vi "EOL CAN_FBL_S19 C70.vi"(8 "Error in":errorcluster, 10 "Read Session in":refnum<k21>, 11 "Write Session in":refnum<k21>) -> (1 "Motor Calibration Response":string, 2 "debug log":string[][](array[string]), 3 "Response Good?":bool)   [LabVIEW 2018]
uses:
  <vilib>/xnet/xnet.llb/XNET Frame CAN.ctl
  <vilib>/xnet/xnet.llb/XNET Frame Type CAN.ctl
panel:
  out "Rx Data":u8[](array[numeric])
  out "Error out":errorcluster
  in  "Retries":i32=2
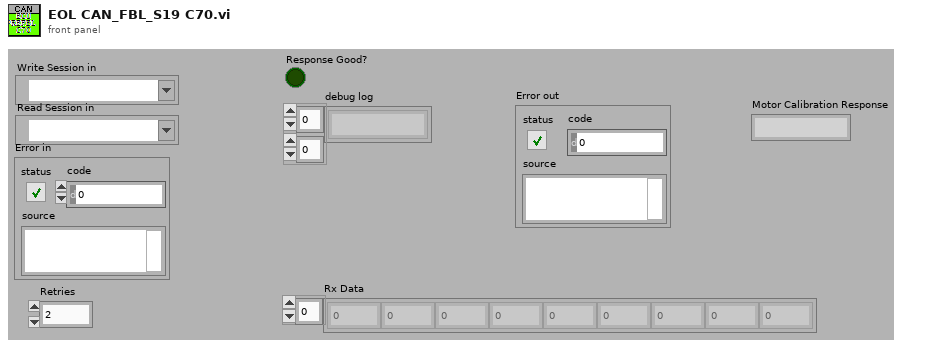
[diagram p1: front panel]
types:
  T1 = cluster{"Write Session in":refnum<k21>, "Read Session in":refnum<k21>, "Error in":errorcluster, "Rx Arbitration Id":u32, "Retry Counter":i32, "TxRx Data":string[][], "Message Start Timer":u32, "Message Wait Timer":i32, "Response Good?":bool, "Rx Data":u8[]}
  T2 = typedef "XNET Frame CAN.ctl" = cluster{"timestamp":timestamp, "payload":u8[], "identifier":u32, "type":T3, "extended?":bool, "echo?":bool}
  T3 = typedef "XNET Frame Type CAN.ctl" = u8
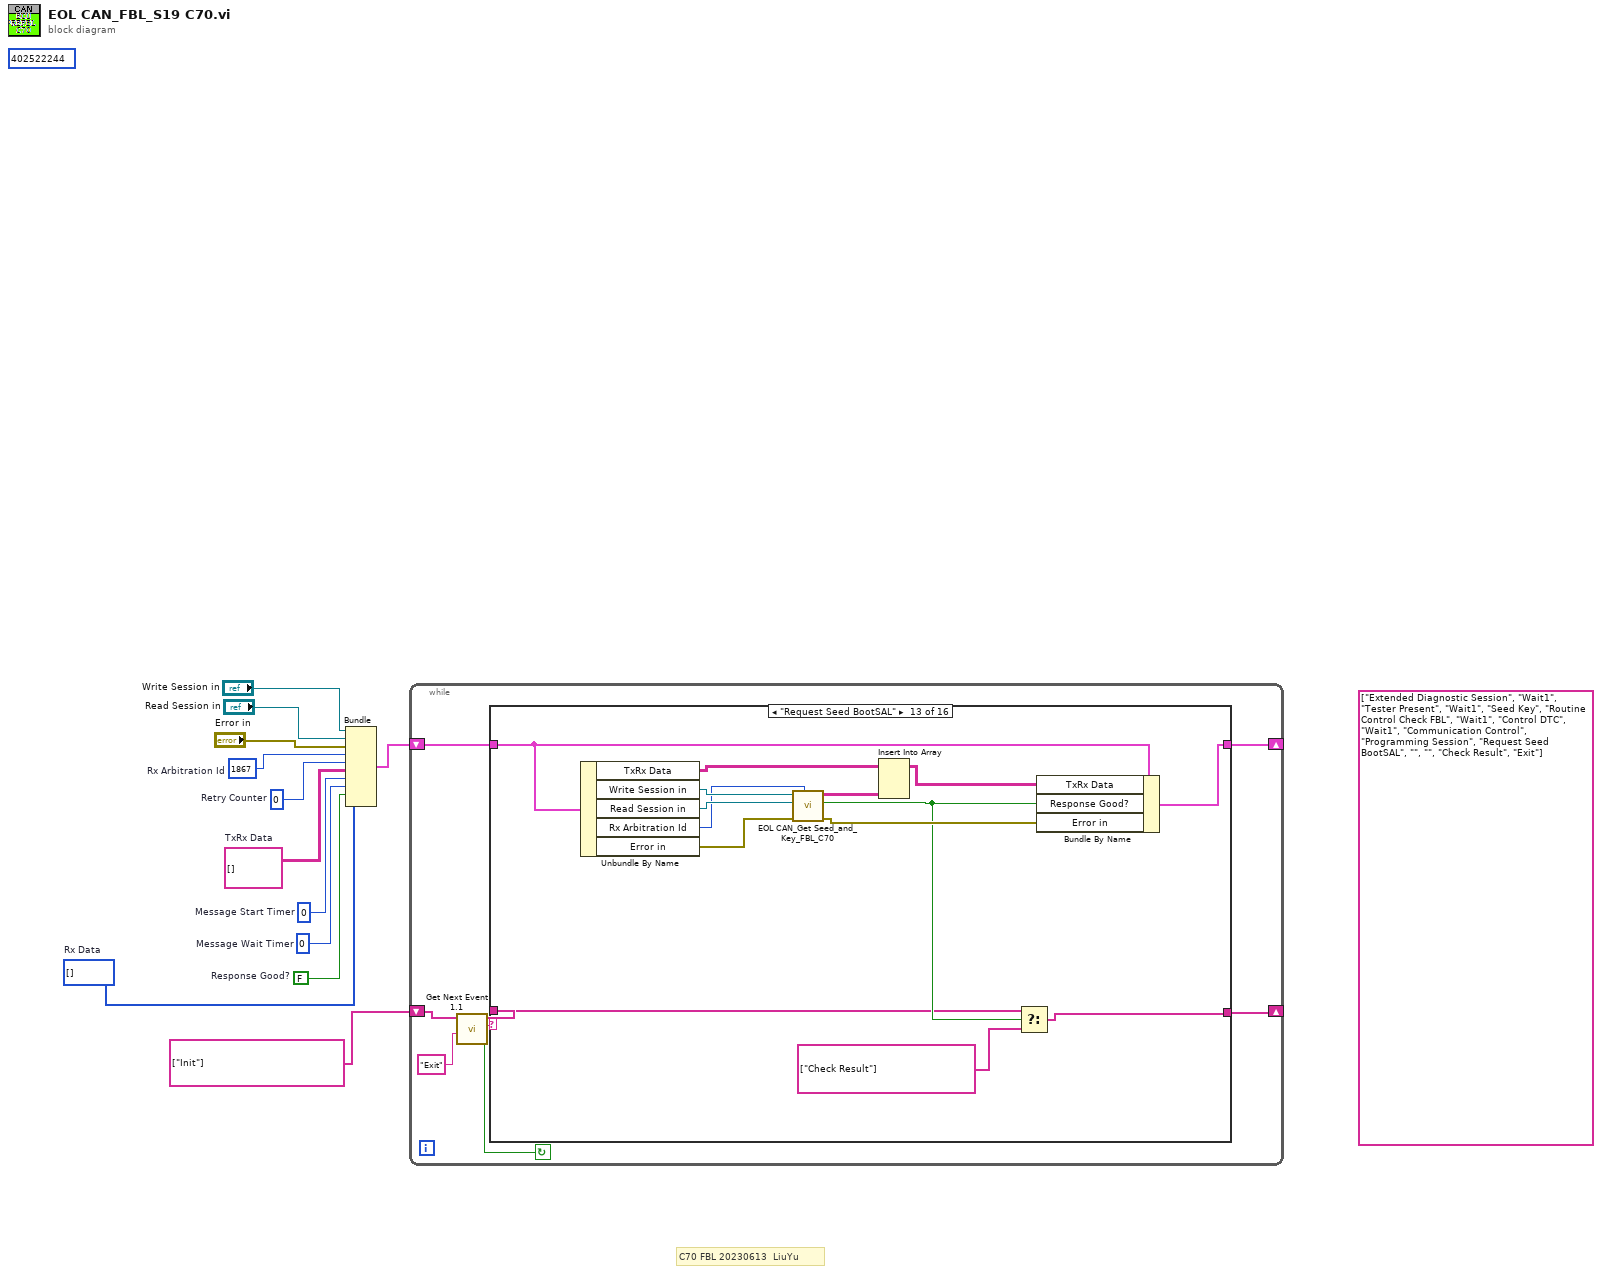
[diagram p0: block diagram]
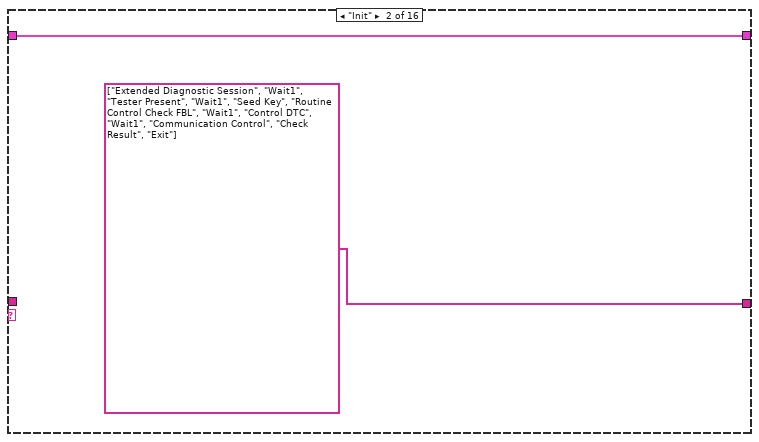
[diagram p3: hidden frame]
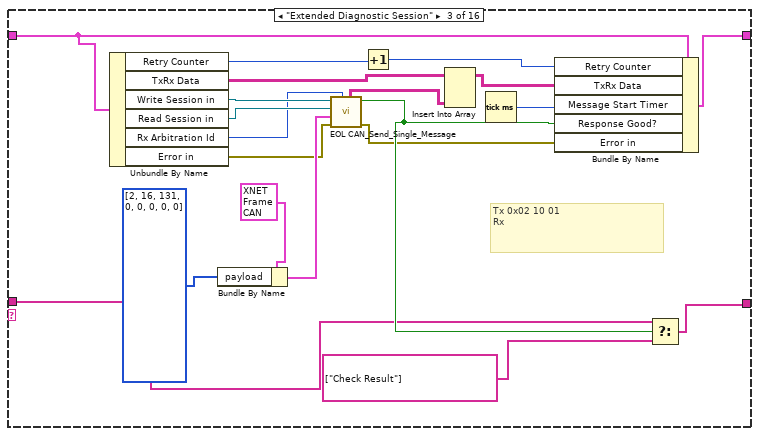
[diagram p4: hidden frame]
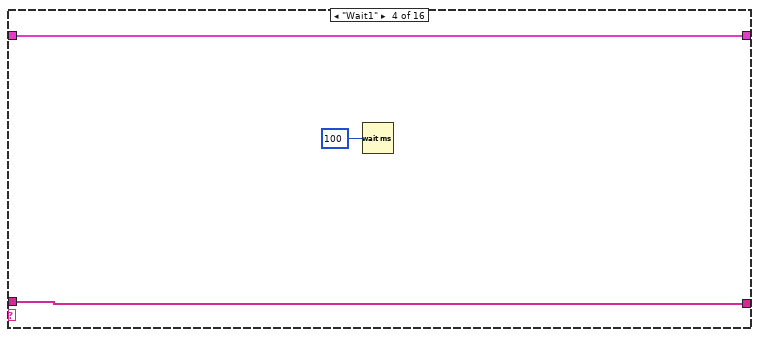
[diagram p5: hidden frame]
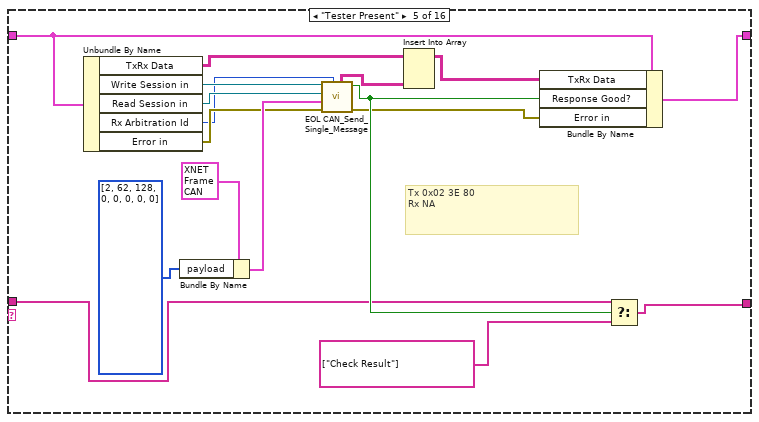
[diagram p6: hidden frame]
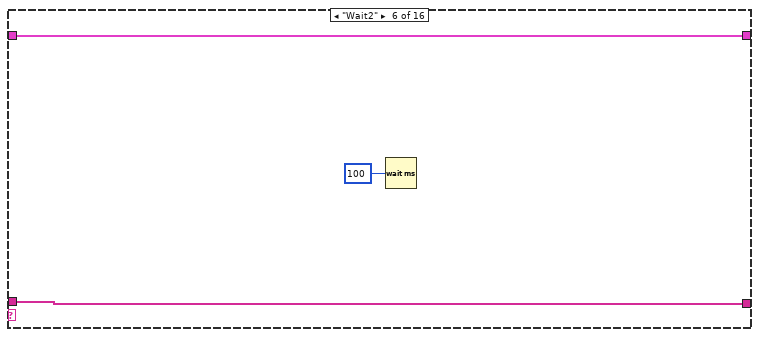
[diagram p7: hidden frame]
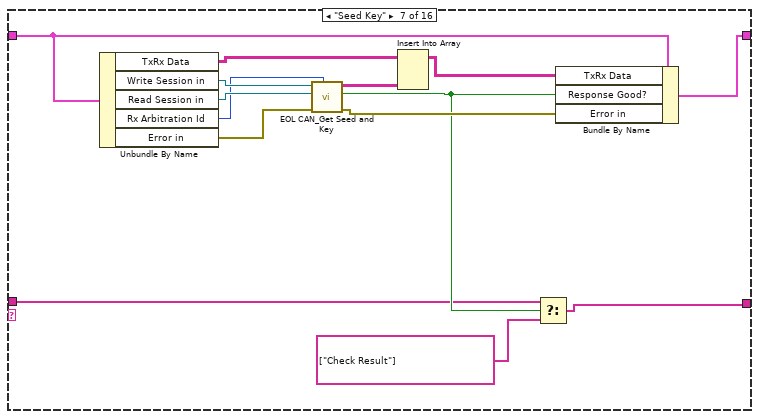
[diagram p8: hidden frame]
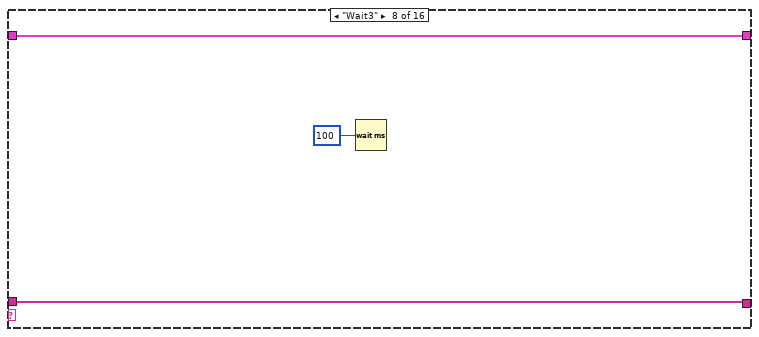
[diagram p9: hidden frame]
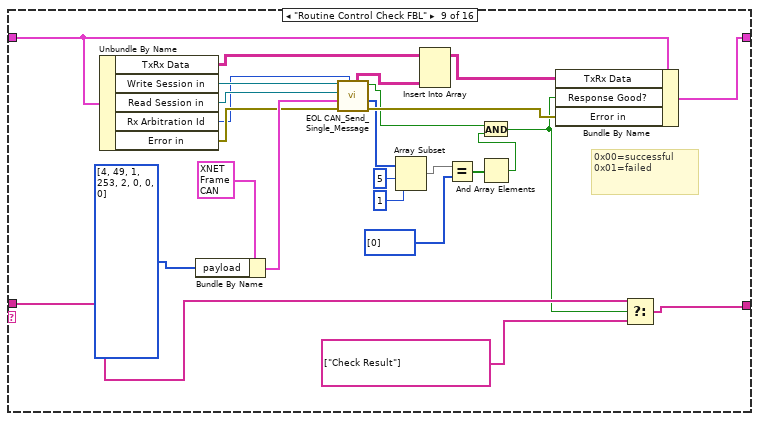
[diagram p10: hidden frame]
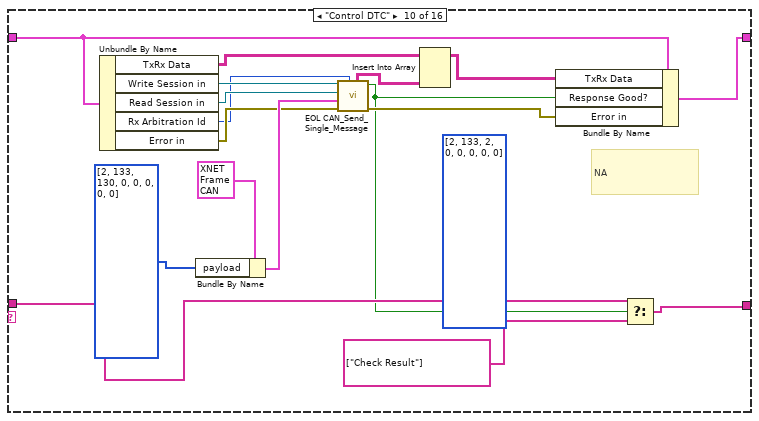
[diagram p11: hidden frame]
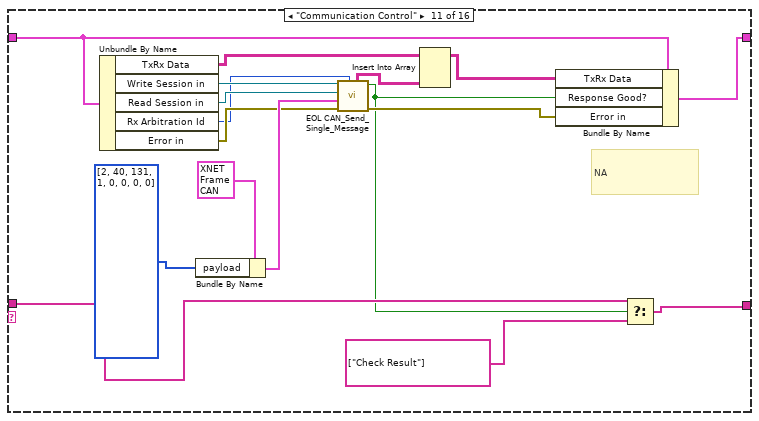
[diagram p12: hidden frame]
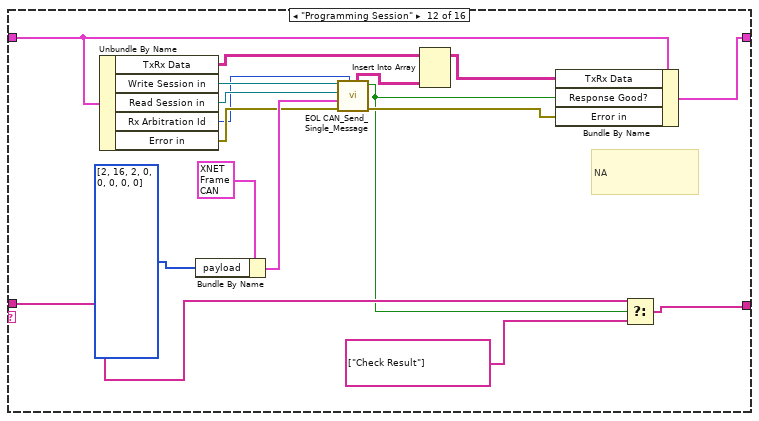
[diagram p13: hidden frame]
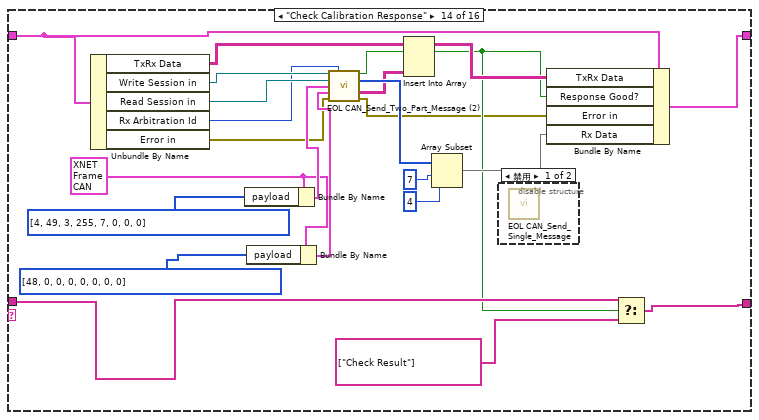
[diagram p14: hidden frame]
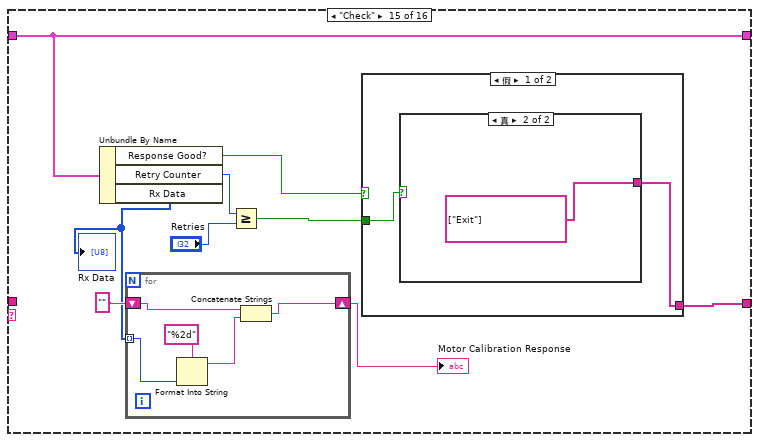
[diagram p16: hidden frame]
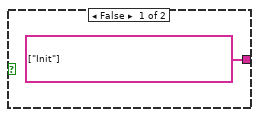
[diagram p17: hidden frame]
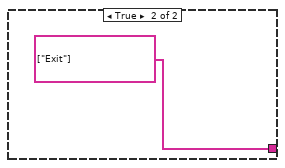
[diagram p18: hidden frame]
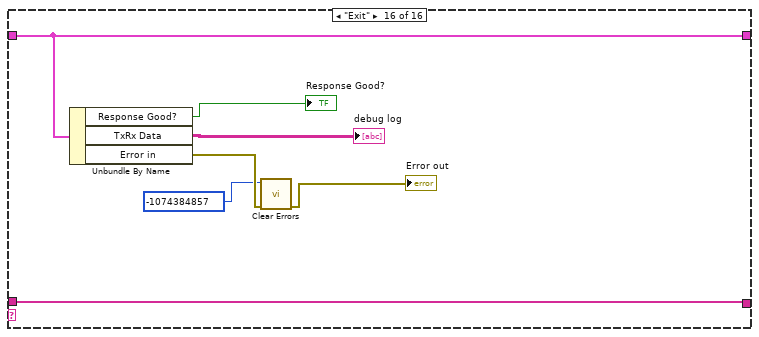
[diagram p19: hidden frame]
diagram:
  w1 = u8[] []  # Rx Data
  w2 = u32 1867  # Rx Arbitration Id
  (unwired) string[] ["Extended Diagnostic Session", "Wait1", "Tester Present", "Wait1", "Seed Key", "Routine Control Check FBL", "Wait1", "Control DTC", "Wait1", "Communication Control", "Programming Session", "Request Seed BootSAL", "", "", "Check Result", "Exit"] ("event queue out")
  w3 = FALSE  # Response Good?
  w4 = 0  # Message Wait Timer
  w5 = u32 0  # Message Start Timer
  w6 = string[][] []  # TxRx Data
  w7 = 0  # Retry Counter
  (unwired) u32 402522244 ("Rx Arbitration Id")
  # "C70 FBL 20230613  LiuYu"
  n1 = Bundle("Write Session in"="Write Session in", "Read Session in"="Read Session in", "Error in"="Error in", "Rx Arbitration Id"=w2, "Retry Counter"=w7, "TxRx Data"=w6, "Message Start Timer"=w5, "Message Wait Timer"=w4, "Response Good?"=w3, "Rx Data"=w1) -> (w8:T1)  [unwired: 1 in]
  n2 = while {
    shift-right: [w13] -> _
    shift-left: string[] ["Init"] -> [w20]
    shift-right: [w15] -> _
    shift-left: w8 -> [w14]
    stop <- w18 continue-if-true
    n3 = call "Get Next Event 1.1.vi"("Exit Event"="Exit", "event queue in"=w20) -> ("Condition (Exit:F)"=w18:bool, "next event"=w17:string, "event queue out"=w16:string[])  [unwired: 6 in, 1 out]
    n4 = case shown="\"Request Seed BootSAL\"" w17 {
      tunnel: w16 -> [w21 _ w25 w46 w48 w65 w70 w82 w96 w113 w130 w147 w163 w191 _ w219]
      tunnel: [w22 w24 w36 w45 w63 w66 w80 w83 w97 w114 w131 w148 w173 w192 w201 w218] -> w15
      tunnel: w14 -> [w22 w24 w37 w45 w64 w66 w81 w83 w98 w115 w132 w149 w174 w193 w201 w218]
      tunnel: [w21 string[] ["Extended Diagnostic Session", "Wait1", "Tester Present", "Wait1", "Seed Key", "Routine Control Check FBL", "Wait1", "Control DTC", "Wait1", "Communication Control", "Check Result", "Exit"] ("event queue out") w27 w46 w50 w65 w69 w82 w95 w112 w129 w146 w162 w190 w205 w219] -> w13
      frame "Error", Default {
      }
      frame "Init" {
      }
      frame "Extended Diagnostic Session" {
        # "Tx 0x02 10 01\nRx"
        n5 = Unbundle By Name(w37) -> ("Retry Counter"=w34:i32, "TxRx Data"=w33:string[][], "Write Session in"=w44:refnum<k21>, "Read Session in"=w43:refnum<k21>, "Rx Arbitration Id"=w42:u32, "Error in"=w38:errorcluster)
        n6 = Bundle By Name(cluster=T2 {"timestamp"=timestamp(0 s since 1904-01-01), "payload"=[2, 39, 3, 85, 85, 85, 85, 85], "identifier"=1859, "type"=8, "extended?"=FALSE, "echo?"=FALSE} ("Tx CAN frame"), "payload"=u8[] [2, 16, 131, 0, 0, 0, 0, 0] ("Transmit Data 2")) -> (w39:T2)
        n7 = call "EOL CAN_Send_Single_Message.vi"("Rx Arbitration Id"=w42, "Error in"=w38, "Tx CAN frame"=w39, "Read Session in"=w43, "Write Session in"=w44) -> ("Error out"=w26:errorcluster, "Response Good?"=w29:bool, "TxRx Data"=w32:string[][])  [unwired: 2 in, 2 out]
        n8 = Increment(x=w34) -> (x+1=w35:i32)
        n9 = Insert Into Array(array=w33, new element=w32) -> (w31:string[][])  [unwired: 2 in]
        n10 = Tick Count (ms)() -> (millisecond timer value=w30:u32)
        n11 = Bundle By Name(cluster=w37, "Retry Counter"=w35, "TxRx Data"=w31, "Message Start Timer"=w30, "Response Good?"=w29, "Error in"=w26) -> (w36:T1)
        n12 = Select(t=w25, s=w29, f=string[] ["Check Result"] ("event queue out")) -> (s? t:f=w27:string[])
      }
      frame "Wait1" {
        n13 = Wait (ms)(milliseconds to wait=u32 100) -> ()  [unwired: 1 out]
      }
      frame "Tester Present" {
        # "Tx 0x02 3E 80\nRx NA"
        n14 = Unbundle By Name(w64) -> ("TxRx Data"=w55:string[][], "Write Session in"=w62:refnum<k21>, "Read Session in"=w61:refnum<k21>, "Rx Arbitration Id"=w56:u32, "Error in"=w57:errorcluster)
        n15 = Bundle By Name(cluster=T2 {"timestamp"=timestamp(0 s since 1904-01-01), "payload"=[2, 39, 3, 85, 85, 85, 85, 85], "identifier"=1859, "type"=8, "extended?"=FALSE, "echo?"=FALSE} ("Tx CAN frame"), "payload"=u8[] [2, 62, 128, 0, 0, 0, 0, 0] ("Transmit Data 2")) -> (w58:T2)
        n16 = call "EOL CAN_Send_Single_Message.vi"("Rx Arbitration Id"=w56, "Error in"=w57, "Tx CAN frame"=w58, "Read Session in"=w61, "Write Session in"=w62) -> ("Error out"=w49:errorcluster, "Response Good?"=w52:bool, "TxRx Data"=w54:string[][])  [unwired: 2 in, 2 out]
        n17 = Insert Into Array(array=w55, new element=w54) -> (w53:string[][])  [unwired: 2 in]
        n18 = Bundle By Name(cluster=w64, "TxRx Data"=w53, "Response Good?"=w52, "Error in"=w49) -> (w63:T1)
        n19 = Select(t=w48, s=w52, f=string[] ["Check Result"] ("event queue out")) -> (s? t:f=w50:string[])
      }
      frame "Wait2" {
        n20 = Wait (ms)(milliseconds to wait=u32 100) -> ()  [unwired: 1 out]
      }
      frame "Seed Key" {
        n21 = Unbundle By Name(w81) -> ("TxRx Data"=w74:string[][], "Write Session in"=w79:refnum<k21>, "Read Session in"=w78:refnum<k21>, "Rx Arbitration Id"=w77:u32, "Error in"=w76:errorcluster)
        n22 = call "EOL CAN_Get Seed and Key.vi"("Rx Arbitration Id"=w77, "Error in"=w76, "Read Session in"=w78, "Write Session in"=w79) -> ("Error out"=w75:errorcluster, "Response Good?"=w71:bool, "TxRx Data"=w73:string[][])  [unwired: 5 in]
        n23 = Insert Into Array(array=w74, new element=w73) -> (w72:string[][])  [unwired: 2 in]
        n24 = Select(t=w70, s=w71, f=string[] ["Check Result"] ("event queue out")) -> (s? t:f=w69:string[])
        n25 = Bundle By Name(cluster=w81, "TxRx Data"=w72, "Response Good?"=w71, "Error in"=w75) -> (w80:T1)
      }
      frame "Wait3" {
        n26 = Wait (ms)(milliseconds to wait=u32 100 ("等待时间（毫秒）")) -> ()  [unwired: 1 out]
      }
      frame "Routine Control Check FBL" {
        # "0x00=successful\n0x01=failed"
        n27 = Unbundle By Name(w98) -> ("TxRx Data"=w103:string[][], "Write Session in"=w109:refnum<k21>, "Read Session in"=w108:refnum<k21>, "Rx Arbitration Id"=w104:u32, "Error in"=w105:errorcluster)
        n28 = Bundle By Name(cluster=T2 {"timestamp"=timestamp(0 s since 1904-01-01), "payload"=[2, 39, 3, 85, 85, 85, 85, 85], "identifier"=1859, "type"=8, "extended?"=FALSE, "echo?"=FALSE} ("Tx CAN frame"), "payload"=u8[] [4, 49, 1, 253, 2, 0, 0, 0] ("Transmit Data 2")) -> (w106:T2)
        n29 = call "EOL CAN_Send_Single_Message.vi"("Rx Arbitration Id"=w104, "Error in"=w105, "Tx CAN frame"=w106, "Read Session in"=w108, "Write Session in"=w109) -> ("Error out"=w99:errorcluster, "Rx Message"=w93:u8[], "Response Good?"=w87:bool, "TxRx Data"=w102:string[][])  [unwired: 2 in, 1 out]
        n30 = Array Subset(array=w93, index=5 ("索引"), length=1 ("长度")) -> (w90:u8[])
        n31 = Insert Into Array(array=w103, new element=w102) -> (w101:string[][])  [unwired: 2 in]
        n32 = Equal?(x=w90, y=u8[] [0]) -> (x = y?=w88:bool[])
        n33 = And Array Elements(Boolean array=w88) -> (logical AND=w86:bool)
        n34 = And(x=w87, y=w86) -> (x .and. y?=w85:bool)
        n35 = Bundle By Name(cluster=w98, "TxRx Data"=w101, "Response Good?"=w85, "Error in"=w99) -> (w97:T1)
        n36 = Select(t=w96, s=w85, f=string[] ["Check Result"] ("event queue out")) -> (s? t:f=w95:string[])
      }
      frame "Control DTC" {
        (unwired) u8[] [2, 133, 2, 0, 0, 0, 0, 0] ("Transmit Data 2")
        # "NA"
        n37 = Unbundle By Name(w115) -> ("TxRx Data"=w120:string[][], "Write Session in"=w126:refnum<k21>, "Read Session in"=w125:refnum<k21>, "Rx Arbitration Id"=w121:u32, "Error in"=w122:errorcluster)
        n38 = Bundle By Name(cluster=T2 {"timestamp"=timestamp(0 s since 1904-01-01), "payload"=[2, 39, 3, 85, 85, 85, 85, 85], "identifier"=1859, "type"=8, "extended?"=FALSE, "echo?"=FALSE} ("Tx CAN frame"), "payload"=u8[] [2, 133, 130, 0, 0, 0, 0, 0] ("Transmit Data 2")) -> (w123:T2)
        n39 = call "EOL CAN_Send_Single_Message.vi"("Rx Arbitration Id"=w121, "Error in"=w122, "Tx CAN frame"=w123, "Read Session in"=w125, "Write Session in"=w126) -> ("Error out"=w116:errorcluster, "Response Good?"=w110:bool, "TxRx Data"=w119:string[][])  [unwired: 2 in, 2 out]
        n40 = Insert Into Array(array=w120, new element=w119) -> (w118:string[][])  [unwired: 2 in]
        n41 = Bundle By Name(cluster=w115, "TxRx Data"=w118, "Response Good?"=w110, "Error in"=w116) -> (w114:T1)
        n42 = Select(t=w113, s=w110, f=string[] ["Check Result"] ("event queue out")) -> (s? t:f=w112:string[])
      }
      frame "Communication Control" {
        # "NA"
        n43 = Unbundle By Name(w132) -> ("TxRx Data"=w137:string[][], "Write Session in"=w143:refnum<k21>, "Read Session in"=w142:refnum<k21>, "Rx Arbitration Id"=w138:u32, "Error in"=w139:errorcluster)
        n44 = Bundle By Name(cluster=T2 {"timestamp"=timestamp(0 s since 1904-01-01), "payload"=[2, 39, 3, 85, 85, 85, 85, 85], "identifier"=1859, "type"=8, "extended?"=FALSE, "echo?"=FALSE} ("Tx CAN frame"), "payload"=u8[] [2, 40, 131, 1, 0, 0, 0, 0] ("Transmit Data 2")) -> (w140:T2)
        n45 = call "EOL CAN_Send_Single_Message.vi"("Rx Arbitration Id"=w138, "Error in"=w139, "Tx CAN frame"=w140, "Read Session in"=w142, "Write Session in"=w143) -> ("Error out"=w133:errorcluster, "Response Good?"=w127:bool, "TxRx Data"=w136:string[][])  [unwired: 2 in, 2 out]
        n46 = Insert Into Array(array=w137, new element=w136) -> (w135:string[][])  [unwired: 2 in]
        n47 = Bundle By Name(cluster=w132, "TxRx Data"=w135, "Response Good?"=w127, "Error in"=w133) -> (w131:T1)
        n48 = Select(t=w130, s=w127, f=string[] ["Check Result"] ("event queue out")) -> (s? t:f=w129:string[])
      }
      frame "Programming Session" {
        # "NA"
        n49 = Unbundle By Name(w149) -> ("TxRx Data"=w154:string[][], "Write Session in"=w160:refnum<k21>, "Read Session in"=w159:refnum<k21>, "Rx Arbitration Id"=w155:u32, "Error in"=w156:errorcluster)
        n50 = Bundle By Name(cluster=T2 {"timestamp"=timestamp(0 s since 1904-01-01), "payload"=[2, 39, 3, 85, 85, 85, 85, 85], "identifier"=1859, "type"=8, "extended?"=FALSE, "echo?"=FALSE} ("Tx CAN frame"), "payload"=u8[] [2, 16, 2, 0, 0, 0, 0, 0] ("Transmit Data 2")) -> (w157:T2)
        n51 = call "EOL CAN_Send_Single_Message.vi"("Rx Arbitration Id"=w155, "Error in"=w156, "Tx CAN frame"=w157, "Read Session in"=w159, "Write Session in"=w160) -> ("Error out"=w150:errorcluster, "Response Good?"=w144:bool, "TxRx Data"=w153:string[][])  [unwired: 2 in, 2 out]
        n52 = Insert Into Array(array=w154, new element=w153) -> (w152:string[][])  [unwired: 2 in]
        n53 = Bundle By Name(cluster=w149, "TxRx Data"=w152, "Response Good?"=w144, "Error in"=w150) -> (w148:T1)
        n54 = Select(t=w147, s=w144, f=string[] ["Check Result"] ("event queue out")) -> (s? t:f=w146:string[])
      }
      frame "Request Seed BootSAL" {
        n55 = Unbundle By Name(w174) -> ("TxRx Data"=w167:string[][], "Write Session in"=w172:refnum<k21>, "Read Session in"=w171:refnum<k21>, "Rx Arbitration Id"=w170:u32, "Error in"=w169:errorcluster)
        n56 = call "EOL CAN_Get Seed_and_Key_FBL_C70.vi"("Rx Arbitration Id"=w170, "Error in"=w169, "Read Session in"=w171, "Write Session in"=w172) -> ("Error out"=w168:errorcluster, "Response Good?"=w164:bool, "TxRx Data"=w166:string[][])  [unwired: 5 in]
        n57 = Insert Into Array(array=w167, new element=w166) -> (w165:string[][])  [unwired: 2 in]
        n58 = Select(t=w163, s=w164, f=string[] ["Check Result"] ("event queue out")) -> (s? t:f=w162:string[])
        n59 = Bundle By Name(cluster=w174, "TxRx Data"=w165, "Response Good?"=w164, "Error in"=w168) -> (w173:T1)
      }
      frame "Check Calibration Response" {
        w185 = T2 {"timestamp"=timestamp(0 s since 1904-01-01), "payload"=[2, 39, 3, 85, 85, 85, 85, 85], "identifier"=1859, "type"=8, "extended?"=FALSE, "echo?"=FALSE} ("Tx CAN frame")
        n60 = Unbundle By Name(w193) -> ("TxRx Data"=w196:string[][], "Write Session in"=w181:refnum<k21>, "Read Session in"=w182:refnum<k21>, "Rx Arbitration Id"=w180:u32, "Error in"=w176:errorcluster)
        n61 = Bundle By Name(cluster=w185, "payload"=u8[] [4, 49, 3, 255, 7, 0, 0, 0] ("Transmit Data 2")) -> (w186:T2)
        n62 = Bundle By Name(cluster=w185, "payload"=u8[] [48, 0, 0, 0, 0, 0, 0, 0] ("Transmit Data")) -> (w183:T2)
        n63 = call "EOL CAN_Send_Two_Part_Message (2).vi"("Write Session in"=w181, "Rx Arbitration Id"=w180, "Read Session in"=w182, "Tx CAN frame 1"=w186, "Tx CAN frame 2"=w183, "error in (no error)"=w176) -> ("Response Good?"=w178:bool, "Rx Data"=w179:u8[], "TxRx Data"=w177:string[][], "error out"=w175:errorcluster)  [unwired: 6 in]
        n64 = Insert Into Array(array=w196, new element=w177) -> (w195:string[][])  [unwired: 2 in]
        n65 = Array Subset(array=w179, index=7 ("索引"), length=4 ("长度")) -> (w187:u8[])
        n66 = disable-structure shown="禁用" {
          frame Disabled {
            n67 = call "EOL CAN_Send_Single_Message.vi"() -> ()  [unwired: 7 in, 5 out]
          }
          frame Enabled {
          }
        }
        n68 = Bundle By Name(cluster=w193, "TxRx Data"=w195, "Response Good?"=w178, "Error in"=w175, "Rx Data"=w187) -> (w192:T1)
        n69 = Select(t=w191, s=w178, f=string[] ["Check Result"] ("event queue out")) -> (s? t:f=w190:string[])
      }
      frame "Check" {
        n70 = Unbundle By Name(w201) -> ("Response Good?"=w206:bool, "Retry Counter"=w204:i32, "Rx Data"=w198:u8[])
        "Rx Data" <- w198
        n71 = for {
          tunnel: w198 -> [w210] mode=indexing
          shift-right: [w207] -> w199
          shift-left: "" -> [w208]
          n72 = Format Into String(format string="%2d" ("格式字符串"), w210) -> (resulting string=w209:string)  [unwired: 2 in, 1 out]
          n73 = Concatenate Strings(w208, w209) -> (w207:string)
        }
        "Motor Calibration Response" <- w199
        n74 = Greater Or Equal?(x=w204, y="Retries") -> (x >= y?=w202:bool)
        n75 = case shown="假" w206 {
          tunnel: [w212 string[] ["Exit"] ("event queue out")] -> w205
          tunnel: w202 -> [w213 _]
          frame False {
            n76 = case shown="真" w213 {
              tunnel: [string[] ["Init"] ("event queue out") string[] ["Exit"] ("event queue out")] -> w212
              frame False {
              }
              frame True {
              }
            }
          }
          frame True {
          }
        }
      }
      frame "Exit" {
        n77 = Unbundle By Name(w218) -> ("Response Good?"=→"Response Good?":bool, "TxRx Data"=→"debug log":string[][], "Error in"=w221:errorcluster)
        n78 = call <vilib>:"Clear Errors.vi"("error in (no error)"=w221, "specific error code to clear (0: all)"=-1074384857) -> ("error out"=→"Error out":errorcluster)  [unwired: 4 in, 1 out]
      }
    }
  }
